vi "NMEA_Coord To Decimal Degrees.vi"(6 "Longitude-Direction":T1=enum."East", 7 "Latitude-Direction":T2=enum."North", 9 "Longitude":dbl caption="DDMM.MMMMM format" format="%0.4f [long]", 10 "Latitude":dbl caption="DDMM.MMMMM format" format="%.04f [lat]") -> (1 "Longitude":dbl format="%0.4f [long]", 2 "Latitude":dbl format="%.04f [lat]")   [LabVIEW 2021, in "NMEA_GPS Ublox M8N.lvlib"]
uses:
  NMEA_GPS Ublox M8N.lvlib
  NMEA_Latitude Direction.ctl
  NMEA_Longitude Direction.ctl
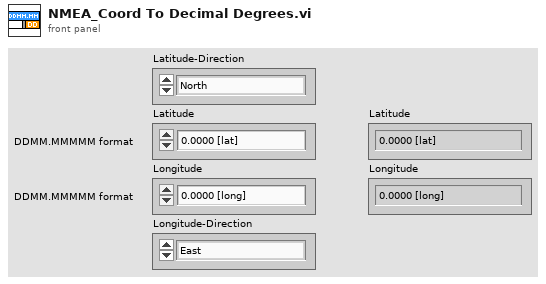
[diagram p1: front panel]
types:
  T1 = typedef "NMEA_GPS Ublox M8N.lvlib/NMEA_Longitude Direction.ctl" = enum16{"", "East", "West"}
  T2 = typedef "NMEA_GPS Ublox M8N.lvlib/NMEA_Latitude Direction.ctl" = enum16{"", "North", "South"}
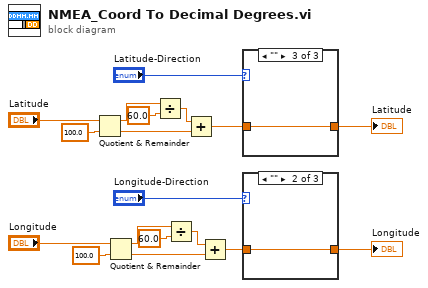
[diagram p0: block diagram]
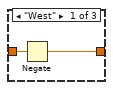
[diagram p2: hidden frame]
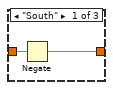
[diagram p4: hidden frame]
diagram:
  n1 = Quotient & Remainder(x="Latitude", y=100.0) -> (x-y*floor(x/y)=w18:dbl, floor(x/y)=w16:dbl)
  n2 = Quotient & Remainder(x="Longitude", y=100.0) -> (x-y*floor(x/y)=w9:dbl, floor(x/y)=w11:dbl)
  n3 = Divide(x=w18, y=60.0) -> (x/y=w15:dbl)
  n4 = Divide(x=w9, y=60.0) -> (x/y=w12:dbl)
  n5 = Add(x=w15, y=w16) -> (x+y=w14:dbl)
  n6 = Add(x=w12, y=w11) -> (x+y=w13:dbl)
  n7 = case shown="\"\"" "Latitude-Direction" {
    tunnel: w14 -> [w20 w21 w22]
    tunnel: [w19 w21 w22] -> w2
    frame "South" {
      n8 = Negate(x=w20) -> (-x=w19:dbl)
    }
    frame "North" {
    }
    frame "" {
    }
  }
  "Latitude" <- w2
  n9 = case shown="\"\"" "Longitude-Direction" {
    tunnel: w13 -> [w24 w25 w26]
    tunnel: [w23 w25 w26] -> w1
    frame "West" {
      n10 = Negate(x=w24) -> (-x=w23:dbl)
    }
    frame "" {
    }
    frame "East" {
    }
  }
  "Longitude" <- w1
